vi "Add Tag.vi"(7 "ID":u32, 8 "error in (no error)":errorcluster, 10 "Tag Value":refnum<class "Basic Type.lvclass">, 11 "Message in":refnum<class "Raw Message.lvclass">) -> (0 "error out":errorcluster, 3 "Message out":refnum<class "Raw Message.lvclass">)   [LabVIEW 2020, in "Protobuf RAW.lvlib" / "Raw Message.lvclass"]
uses:
  Raw Message.lvclass
  Tag/Basic Type.lvclass
  Raw Message.lvclass/Raw Message.ctl
  <vilib>/Utility/miscctls.llb/LVMapReplaceAction.ctl
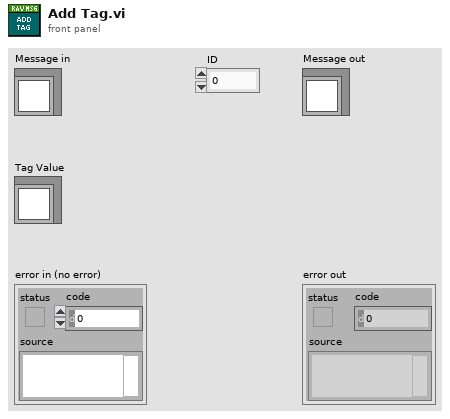
[diagram p1: front panel]
types:
  T1 = typedef "LVMapReplaceAction.ctl" = enum32{"Modify Entry only if found", "Add or Modify Entry", "Delete Entry"}
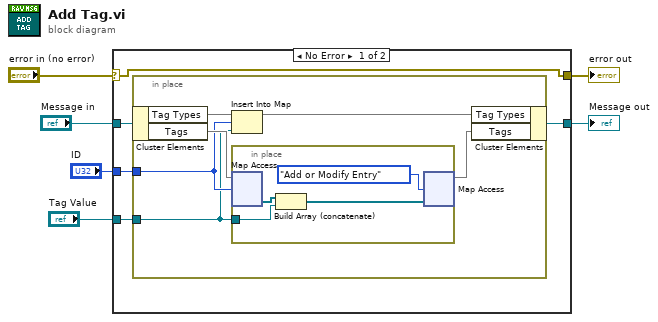
[diagram p0: block diagram]
diagram:
  n1 = case shown="No Error" "error in (no error)" {
    selector: "error in (no error)" -> [w10 w23]
    tunnel: [w10 w23] -> w5
    tunnel: [w9 w22] -> w3
    tunnel: "Message in" -> [w11 w22]
    tunnel: "ID" -> [w8 _]
    tunnel: "Tag Value" -> [w7 _]
    frame No Error {
      n2 = in-place {
        in-place-border: w8 -> [w13]
        in-place-border: w7 -> [w12]
        n3 = in-place-cluster #1(w11) -> ("Tag Types"=w17:map{u32, refnum<class "Basic Type.lvclass">}, "Tags"=w15:map{u32, refnum<class "Basic Type.lvclass">[]})
        n4 = Insert Into Map(map in=w17, key=w13, value=w12) -> (map out=w16:map{u32, refnum<class "Basic Type.lvclass">})  [unwired: 2 out]
        n5 = in-place {
          in-place-border: w12 -> [w19]
          n6 = in-place-map #2(w15, w13) -> (w21:refnum<class "Basic Type.lvclass">[])  [unwired: 1 in, 1 out]
          n7 = Build Array (concatenate)(w21, w19) -> (w20:refnum<class "Basic Type.lvclass">[])
          n8 = in-place-map #2(w20, LVMapReplaceAction."Add or Modify Entry" ("action")) -> (w14:map{u32, refnum<class "Basic Type.lvclass">[]})  [unwired: 2 out]
        }
        n9 = in-place-cluster #1("Tag Types"=w16, "Tags"=w14) -> (w9:refnum<class "Raw Message.lvclass">)
      }
    }
    frame Error {
    }
  }
  "error out" <- w5
  "Message out" <- w3
